vi "Get INI Data.vi"(8 "error in":errorcluster, 11 "Section":T1) -> (0 "error out":errorcluster, 3 "INI Data":T2(array[cluster]))   [LabVIEW 2019]
uses:
  Controls/Section List.ctl
  Controls/KeyValue.ctl
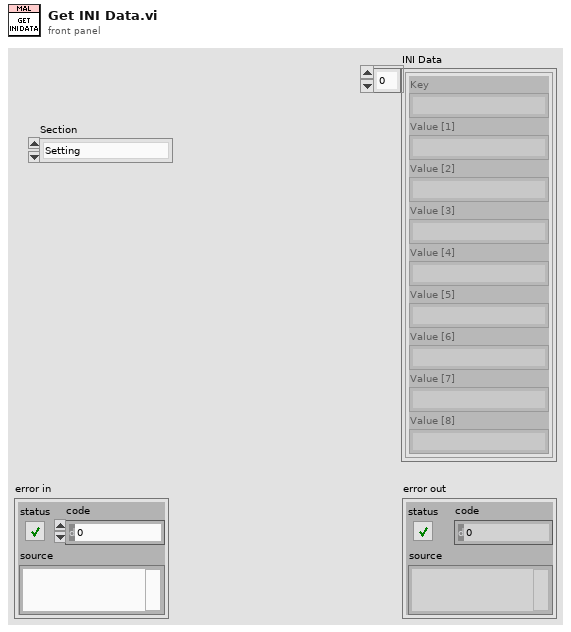
[diagram p1: front panel]
types:
  T1 = typedef "Section List.ctl" = enum16{"Setting", "Instruments", "Digital_Out", "Digital_In", "NI_DMM"}
  T2 = cluster{"Key":string, "Value [1]":string, "Value [2]":string, "Value [3]":string, "Value [4]":string, "Value [5]":string, "Value [6]":string, "Value [7]":string, "Value [8]":string}[]
  T3 = typedef "KeyValue.ctl" = cluster{"Key":string, "Value":string}
  T4 = typedef "MAL.lvlib/INI DataType.ctl" = cluster{"Section":string, "Data":variant}
  T5 = cluster{"string array[0]":string, "string array[1]":string, "string array[2]":string, "string array[3]":string, "string array[4]":string, "string array[5]":string, "string array[6]":string, "string array[7]":string, "string array[8]":string}
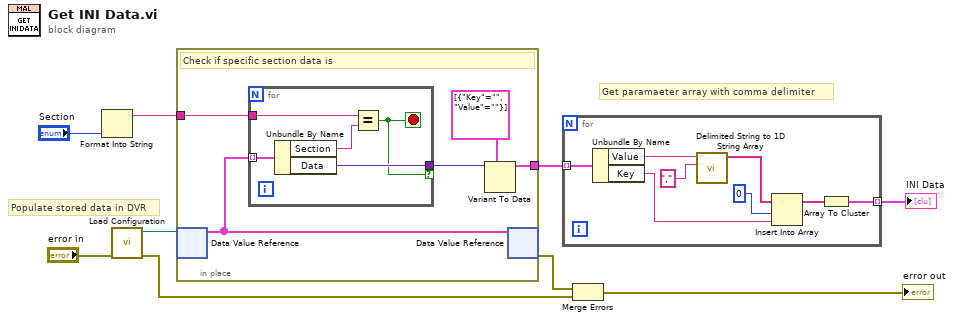
[diagram p0: block diagram]
diagram:
  # "Populate stored data in DVR"
  # "Get paramaeter array with comma delimiter"
  n1 = Format Into String("Section") -> (resulting string=w1:string)  [unwired: 3 in, 1 out]
  n2 = call "Load Configuration.vi"("error in"="error in") -> ("error out"=w9:errorcluster, "Config DVR"=w7:refnum<data-value>)  [unwired: 9 in]
  n3 = in-place {
    in-place-border: [w12] -> w6
    in-place-border: w1 -> [w10]
    # "Check if specific section data is"
    n4 = in-place-dvr #1(w7) -> (w13:T4[])  [unwired: 1 out]
    n5 = for {
      tunnel: w13 -> [w19] mode=indexing
      tunnel: [w17] -> w14 if=w16
      tunnel: w10 -> [w15]
      stop <- w16 stop-if-true
      n6 = Unbundle By Name(w19) -> ("Section"=w18:string, "Data"=w17:variant)
      n7 = Equal?(x=w15, y=w18) -> (x = y?=w16:bool)
    }
    n8 = Variant To Data(type=T3[] [{"Key"="", "Value"=""}], Variant=w14) -> (data=w12:T3[])  [unwired: 1 in, 1 out]
    n9 = in-place-dvr #1(w13) -> (w8:errorcluster)  [unwired: 1 out]
  }
  n10 = for {
    tunnel: w6 -> [w26] mode=indexing
    tunnel: [w20] -> w3 mode=indexing
    n11 = Unbundle By Name(w26) -> ("Value"=w25:string, "Key"=w23:string)
    n12 = call <vilib>:"Delimited String to 1D String Array.vi"("delimiter"=",", "delimited string"=w25) -> ("string array"=w24:string[])  [unwired: 9 in]
    n13 = Insert Into Array(array=w24, index=0, new element=w23) -> (w21:string[])
    n14 = Array To Cluster(array=w21) -> (cluster=w20:T5)
  }
  "INI Data" <- w3
  n15 = Merge Errors(w8, w9) -> (→"error out":errorcluster)
